vi "SpreadsheetFGV2_Improvements.vi"(0 "Student ID":i32, 1 "State Options":T4, 2 "Camera Name":refnum<k21> caption="IMAQdx Session", 5 "Message Ref":refnum<vi>, 9 "Front Panel References":refnum<vi>[](array[refnum]), 11 "Error In":errorcluster) -> (3 "Time Stamp Out":timestamp=timestamp(3628529847.18708 s since 1904-01-01), 4 "Message":string="Shut Down", 6 "Names":string[](array[string]), 8 "Output 2D Data":string[][](array[string])=[["Full Name", "Check In", "Check Out", "Checked In?", "Hours", "Minutes", "Seconds", "Total Seconds", "Col1", "Col2", "Col3", "Record ID (ref)", "Related Season Log"], ["Aden Lok", "", "", "FALSE", "", "", "", "", "0", "0", "0", "167", "239"], ["Aidan Egan", "", "", "FALSE", "", "", "", "", "0", "0", "0", "12", "240"], ["Alejandro Magadan", "12/24/2018 3:47:18 PM", "12/24/2018 3:53:19 PM", "FALSE", "15", "47", "18", "361", "0", "0", "0", "166", "241"], ["Alessandro Carleton", "", "", "FALSE", "", "", "", "", "0", "0", "0", "165", "242"], ["Amaan Ali", "", "", "FALSE", "", "", "", "", "0", "0", "0", "168", "243"], ["An Ngo", "", "", "FALSE", "", "", "", "", "0", "0", "0", "163", "244"], ["Avery Jennings", "", "", "FALSE", "", "", "", "", "0", "0", "0", "102", "245"], ["Brendan Webb", "12/24/2018 3:39:05 PM", "12/24/2018 3:53:19 PM", "FALSE", "15", "39", "05", "854", "0", "0", "0", "33", "246"], ["Brendan Byrne", "12/24/2018 3:47:17 PM", "12/24/2018 3:53:19 PM", "FALSE", "15", "47", "17", "362", "0", "0", "0", "169", "247"], ["Charles Jacobson", "12/24/2018 3:47:12 PM", "12/24/2018 3:48:43 PM", "FALSE", "15", "47", "12", "91", "0", "0", "0", "110", "248"], ["Chase Thomas", "", "", "FALSE", "", "", "", "", "0", "0", "0", "24", "249"], ["Christian Davis", "", "", "FALSE", "", "", "", "", "0", "0", "0", "171", "250"], ["Christopher Keith", "", "", "FALSE", "", "", "", "", "0", "0", "0", "170", "251"], ["Colman Gillis", "", "", "FALSE", "", "", "", "", "0", "0", "0", "62", "252"], ["Daniel Murtagh", "12/24/2018 3:38:36 PM", "12/24/2018 3:53:19 PM", "FALSE", "15", "38", "36", "883", "0", "0", "0", "173", "253"], ["Daniel Politano", "", "", "FALSE", "", "", "", "", "0", "0", "0", "175", "254"], ["Donovan Moore", "", "", "FALSE", "", "", "", "", "0", "0", "0", "174", "255"], ["Dyllan Bui", "", "", "FALSE", "", "", "", "", "0", "0", "0", "172", "256"], ["Henry Synnott", "", "", "FALSE", "", "", "", "", "0", "0", "0", "176", "257"], ["Huy GIang", "12/24/2018 3:47:20 PM", "12/24/2018 3:53:19 PM", "FALSE", "15", "47", "20", "359", "0", "0", "0", "177", "258"], ["Isaiah Jean-Fontaine", "", "", "FALSE", "", "", "", "", "0", "0", "0", "178", "259"], ["Jack Duggan", "", "", "FALSE", "", "", "", "", "0", "0", "0", "11", "260"], ["Jack Morris", "", "", "FALSE", "", "", "", "", "0", "0", "0", "181", "261"], ["Jake Monahan", "", "", "FALSE", "", "", "", "", "0", "0", "0", "189", "262"], ["James McEneaney", "", "", "FALSE", "", "", "", "", "0", "0", "0", "180", "263"], ["Jason Murray", "", "", "FALSE", "", "", "", "", "0", "0", "0", "16", "264"], ["Javed Brathwaite", "12/24/2018 3:39:10 PM", "12/24/2018 3:41:41 PM", "FALSE", "15", "39", "10", "151", "0", "0", "0", "72", "265"], ["Jay Siegfried", "", "", "FALSE", "", "", "", "", "0", "0", "0", "73", "266"], ["Jeffrey Chen", "", "", "FALSE", "", "", "", "", "0", "0", "0", "179", "267"], ["Karsten Patzer", "", "12/24/2018 3:53:19 PM", "FALSE", "", "", "", "57199", "0", "0", "0", "182", "268"], ["Liam Walsh", "", "", "FALSE", "", "", "", "", "0", "0", "0", "134", "269"], ["Lucas Hurley", "", "", "FALSE", "", "", "", "", "0", "0", "0", "183", "270"], ["Luke Reid", "", "", "FALSE", "", "", "", "", "0", "0", "0", "93", "271"], ["Maxwell Malamut", "", "", "FALSE", "", "", "", "", "0", "0", "0", "133", "272"], ["Nicholas Hurley", "", "", "FALSE", "", "", "", "", "0", "0", "0", "121", "273"], ["Philip Byrne", "", "", "FALSE", "", "", "", "", "0", "0", "0", "184", "274"], ["Praveen Kalva", "", "", "FALSE", "", "", "", "", "0", "0", "0", "185", "275"], ["Rohan Joshi", "", "", "FALSE", "", "", "", "", "0", "0", "0", "84", "276"], ["Samuel Danby", "", "", "FALSE", "", "", "", "", "0", "0", "0", "9", "277"], ["Thomas Potts", "", "", "FALSE", "", "", "", "", "0", "0", "0", "111", "278"], ["Timmy Tran", "", "", "FALSE", "", "", "", "", "0", "0", "0", "186", "279"], ["Willem Lenig", "", "", "FALSE", "", "", "", "", "0", "0", "0", "188", "280"], ["William Lau", "", "", "FALSE", "", "", "", "", "0", "0", "0", "187", "281"]], 10 "Checked In?":bool, 12 "Cat Points":i32, 13 "Image Out":T2(plugin-control), 14 "Elapsed Time":dbl, 15 "Error Out":errorcluster)   [LabVIEW 2018]
uses:
  Controls/CSVFGVStates.ctl
  <vilib>/userdefined/High Color/IMAQdx.ctl
  Controls/SpreadsheetColumns.ctl
  Controls/ClockType.ctl
  <vilib>/Utility/file.llb/Write Delimited Spreadsheet (string).vi
  <vilib>/Utility/file.llb/Read Delimited Spreadsheet (string).vi
  <vilib>/vision/driver/NI_Vision_Acquisition_Software.lvlib
panel:
  out "IDs":string[](array[string])
  out "headers":string
  out "body":string
  out "Camera Information Array":T1(array[cluster])=[{"Type"=3, "Version"=2, "Flags"=1, "SerialNumberHigh"=2886719754, "SerialNumberLow"=3015254064, "BusType"=1685284983, "InterfaceName"="cam2", "VendorName"="Microsoft® LifeCam Studio(TM)", "ModelName"="", "CameraFileName"="Microsoft® LifeCam Studio(TM)  (#AC0FD90AB3B92030).icd", "CameraAttributeURL"=""}] {"BusType" format="%x"; "SerialNumberLow" format="%.0x"; "SerialNumberHigh" format="%.0x"}
  out "Table List":string[][](array[string])=[["Full Name", "Check In", "Check Out", "Checked In?", "Hours", "Minutes", "Seconds", "Total Seconds", "Col1", "Col2", "Col3", "Record ID (ref)", "Related Season Log"], ["Aden Lok", "", "", "FALSE", "", "", "", "", "0", "0", "0", "167", "239"], ["Aidan Egan", "", "", "FALSE", "", "", "", "", "0", "0", "0", "12", "240"], ["Alejandro Magadan", "12/24/2018 3:47:18 PM", "12/24/2018 3:53:19 PM", "FALSE", "15", "47", "18", "361", "0", "0", "0", "166", "241"], ["Alessandro Carleton", "", "", "FALSE", "", "", "", "", "0", "0", "0", "165", "242"], ["Amaan Ali", "", "", "FALSE", "", "", "", "", "0", "0", "0", "168", "243"], ["An Ngo", "", "", "FALSE", "", "", "", "", "0", "0", "0", "163", "244"], ["Avery Jennings", "", "", "FALSE", "", "", "", "", "0", "0", "0", "102", "245"], ["Brendan Webb", "12/24/2018 3:39:05 PM", "12/24/2018 3:53:19 PM", "FALSE", "15", "39", "05", "854", "0", "0", "0", "33", "246"], ["Brendan Byrne", "12/24/2018 3:47:17 PM", "12/24/2018 3:53:19 PM", "FALSE", "15", "47", "17", "362", "0", "0", "0", "169", "247"], ["Charles Jacobson", "12/24/2018 3:47:12 PM", "12/24/2018 3:48:43 PM", "FALSE", "15", "47", "12", "91", "0", "0", "0", "110", "248"], ["Chase Thomas", "", "", "FALSE", "", "", "", "", "0", "0", "0", "24", "249"], ["Christian Davis", "", "", "FALSE", "", "", "", "", "0", "0", "0", "171", "250"], ["Christopher Keith", "", "", "FALSE", "", "", "", "", "0", "0", "0", "170", "251"], ["Colman Gillis", "", "", "FALSE", "", "", "", "", "0", "0", "0", "62", "252"], ["Daniel Murtagh", "12/24/2018 3:38:36 PM", "12/24/2018 3:53:19 PM", "FALSE", "15", "38", "36", "883", "0", "0", "0", "173", "253"], ["Daniel Politano", "", "", "FALSE", "", "", "", "", "0", "0", "0", "175", "254"], ["Donovan Moore", "", "", "FALSE", "", "", "", "", "0", "0", "0", "174", "255"], ["Dyllan Bui", "", "", "FALSE", "", "", "", "", "0", "0", "0", "172", "256"], ["Henry Synnott", "", "", "FALSE", "", "", "", "", "0", "0", "0", "176", "257"], ["Huy GIang", "12/24/2018 3:47:20 PM", "12/24/2018 3:53:19 PM", "FALSE", "15", "47", "20", "359", "0", "0", "0", "177", "258"], ["Isaiah Jean-Fontaine", "", "", "FALSE", "", "", "", "", "0", "0", "0", "178", "259"], ["Jack Duggan", "", "", "FALSE", "", "", "", "", "0", "0", "0", "11", "260"], ["Jack Morris", "", "", "FALSE", "", "", "", "", "0", "0", "0", "181", "261"], ["Jake Monahan", "", "", "FALSE", "", "", "", "", "0", "0", "0", "189", "262"], ["James McEneaney", "", "", "FALSE", "", "", "", "", "0", "0", "0", "180", "263"], ["Jason Murray", "", "", "FALSE", "", "", "", "", "0", "0", "0", "16", "264"], ["Javed Brathwaite", "12/24/2018 3:39:10 PM", "12/24/2018 3:41:41 PM", "FALSE", "15", "39", "10", "151", "0", "0", "0", "72", "265"], ["Jay Siegfried", "", "", "FALSE", "", "", "", "", "0", "0", "0", "73", "266"], ["Jeffrey Chen", "", "", "FALSE", "", "", "", "", "0", "0", "0", "179", "267"], ["Karsten Patzer", "", "12/24/2018 3:53:19 PM", "FALSE", "", "", "", "57199", "0", "0", "0", "182", "268"], ["Liam Walsh", "", "", "FALSE", "", "", "", "", "0", "0", "0", "134", "269"], ["Lucas Hurley", "", "", "FALSE", "", "", "", "", "0", "0", "0", "183", "270"], ["Luke Reid", "", "", "FALSE", "", "", "", "", "0", "0", "0", "93", "271"], ["Maxwell Malamut", "", "", "FALSE", "", "", "", "", "0", "0", "0", "133", "272"], ["Nicholas Hurley", "", "", "FALSE", "", "", "", "", "0", "0", "0", "121", "273"], ["Philip Byrne", "", "", "FALSE", "", "", "", "", "0", "0", "0", "184", "274"], ["Praveen Kalva", "", "", "FALSE", "", "", "", "", "0", "0", "0", "185", "275"], ["Rohan Joshi", "", "", "FALSE", "", "", "", "", "0", "0", "0", "84", "276"], ["Samuel Danby", "", "", "FALSE", "", "", "", "", "0", "0", "0", "9", "277"], ["Thomas Potts", "", "", "FALSE", "", "", "", "", "0", "0", "0", "111", "278"], ["Timmy Tran", "", "", "FALSE", "", "", "", "", "0", "0", "0", "186", "279"], ["Willem Lenig", "", "", "FALSE", "", "", "", "", "0", "0", "0", "188", "280"], ["William Lau", "", "", "FALSE", "", "", "", "", "0", "0", "0", "187", "281"]]
  out "Table List":string[][](array[string])=[["Full Name", "Check In", "Check Out", "Checked In?", "Hours", "Minutes", "Seconds", "Total Seconds", "Col1", "Col2", "Col3", "Record ID (ref)", "Related Season Log"], ["Aden Lok", "", "", "FALSE", "", "", "", "", "0", "0", "0", "167", "239"], ["Aidan Egan", "", "", "FALSE", "", "", "", "", "0", "0", "0", "12", "240"], ["Alejandro Magadan", "12/24/2018 3:47:18 PM", "", "TRUE", "15", "47", "18", "", "0", "0", "0", "166", "241"], ["Alessandro Carleton", "", "", "FALSE", "", "", "", "", "0", "0", "0", "165", "242"], ["Amaan Ali", "", "", "FALSE", "", "", "", "", "0", "0", "0", "168", "243"], ["An Ngo", "", "", "FALSE", "", "", "", "", "0", "0", "0", "163", "244"], ["Avery Jennings", "", "", "FALSE", "", "", "", "", "0", "0", "0", "102", "245"], ["Brendan Webb", "12/24/2018 3:39:05 PM", "", "TRUE", "15", "39", "05", "", "0", "0", "0", "33", "246"], ["Brendan Byrne", "12/24/2018 3:47:17 PM", "", "TRUE", "15", "47", "17", "", "0", "0", "0", "169", "247"], ["Charles Jacobson", "12/24/2018 3:47:12 PM", "", "TRUE", "15", "47", "12", "", "0", "0", "0", "110", "248"], ["Chase Thomas", "", "", "FALSE", "", "", "", "", "0", "0", "0", "24", "249"], ["Christian Davis", "", "", "FALSE", "", "", "", "", "0", "0", "0", "171", "250"], ["Christopher Keith", "", "", "FALSE", "", "", "", "", "0", "0", "0", "170", "251"], ["Colman Gillis", "", "", "FALSE", "", "", "", "", "0", "0", "0", "62", "252"], ["Daniel Murtagh", "12/24/2018 3:38:36 PM", "", "TRUE", "15", "38", "36", "", "0", "0", "0", "173", "253"], ["Daniel Politano", "", "", "FALSE", "", "", "", "", "0", "0", "0", "175", "254"], ["Donovan Moore", "", "", "FALSE", "", "", "", "", "0", "0", "0", "174", "255"], ["Dyllan Bui", "", "", "FALSE", "", "", "", "", "0", "0", "0", "172", "256"], ["Henry Synnott", "", "", "FALSE", "", "", "", "", "0", "0", "0", "176", "257"], ["Huy GIang", "", "", "FALSE", "", "", "", "", "0", "0", "0", "177", "258"], ["Isaiah Jean-Fontaine", "", "", "FALSE", "", "", "", "", "0", "0", "0", "178", "259"], ["Jack Duggan", "", "", "FALSE", "", "", "", "", "0", "0", "0", "11", "260"], ["Jack Morris", "", "", "FALSE", "", "", "", "", "0", "0", "0", "181", "261"], ["Jake Monahan", "", "", "FALSE", "", "", "", "", "0", "0", "0", "189", "262"], ["James McEneaney", "", "", "FALSE", "", "", "", "", "0", "0", "0", "180", "263"], ["Jason Murray", "", "", "FALSE", "", "", "", "", "0", "0", "0", "16", "264"], ["Javed Brathwaite", "12/24/2018 3:39:10 PM", "12/24/2018 3:41:41 PM", "FALSE", "15", "39", "10", "151", "0", "0", "0", "72", "265"], ["Jay Siegfried", "", "", "FALSE", "", "", "", "", "0", "0", "0", "73", "266"], ["Jeffrey Chen", "", "", "FALSE", "", "", "", "", "0", "0", "0", "179", "267"], ["Karsten Patzer", "", "", "TRUE", "", "", "", "", "0", "0", "0", "182", "268"], ["Liam Walsh", "", "", "FALSE", "", "", "", "", "0", "0", "0", "134", "269"], ["Lucas Hurley", "", "", "FALSE", "", "", "", "", "0", "0", "0", "183", "270"], ["Luke Reid", "", "", "FALSE", "", "", "", "", "0", "0", "0", "93", "271"], ["Maxwell Malamut", "", "", "FALSE", "", "", "", "", "0", "0", "0", "133", "272"], ["Nicholas Hurley", "", "", "FALSE", "", "", "", "", "0", "0", "0", "121", "273"], ["Philip Byrne", "", "", "FALSE", "", "", "", "", "0", "0", "0", "184", "274"], ["Praveen Kalva", "", "", "FALSE", "", "", "", "", "0", "0", "0", "185", "275"], ["Rohan Joshi", "", "", "FALSE", "", "", "", "", "0", "0", "0", "84", "276"], ["Samuel Danby", "", "", "FALSE", "", "", "", "", "0", "0", "0", "9", "277"], ["Thomas Potts", "", "", "FALSE", "", "", "", "", "0", "0", "0", "111", "278"], ["Timmy Tran", "", "", "FALSE", "", "", "", "", "0", "0", "0", "186", "279"], ["Willem Lenig", "", "", "FALSE", "", "", "", "", "0", "0", "0", "188", "280"], ["William Lau", "", "", "FALSE", "", "", "", "", "0", "0", "0", "187", "281"]]
  out "Session Out":T3="cam2"
  out "Checked In":string="FALSE"
  out "all rows":string[][](array[string])=[["Full Name", "Check In", "Check Out", "Checked In?", "Hours", "Minutes", "Seconds", "Total Seconds", "Col1", "Col2", "Col3", "Record ID (ref)", "Related Season Log"], ["Aden Lok", "", "", "FALSE", "", "", "", "", "0", "0", "0", "167", "239"], ["Aidan Egan", "", "", "FALSE", "", "", "", "", "0", "0", "0", "12", "240"], ["Alejandro Magadan", "12/24/2018 3:47:18 PM", "12/24/2018 3:53:19 PM", "FALSE", "15", "47", "18", "361", "0", "0", "0", "166", "241"], ["Alessandro Carleton", "", "", "FALSE", "", "", "", "", "0", "0", "0", "165", "242"], ["Amaan Ali", "", "", "FALSE", "", "", "", "", "0", "0", "0", "168", "243"], ["An Ngo", "", "", "FALSE", "", "", "", "", "0", "0", "0", "163", "244"], ["Avery Jennings", "", "", "FALSE", "", "", "", "", "0", "0", "0", "102", "245"], ["Brendan Webb", "12/24/2018 3:39:05 PM", "12/24/2018 3:53:19 PM", "FALSE", "15", "39", "05", "854", "0", "0", "0", "33", "246"], ["Brendan Byrne", "12/24/2018 3:47:17 PM", "12/24/2018 3:53:19 PM", "FALSE", "15", "47", "17", "362", "0", "0", "0", "169", "247"], ["Charles Jacobson", "12/24/2018 3:47:12 PM", "12/24/2018 3:48:43 PM", "FALSE", "15", "47", "12", "91", "0", "0", "0", "110", "248"], ["Chase Thomas", "", "", "FALSE", "", "", "", "", "0", "0", "0", "24", "249"], ["Christian Davis", "", "", "FALSE", "", "", "", "", "0", "0", "0", "171", "250"], ["Christopher Keith", "", "", "FALSE", "", "", "", "", "0", "0", "0", "170", "251"], ["Colman Gillis", "", "", "FALSE", "", "", "", "", "0", "0", "0", "62", "252"], ["Daniel Murtagh", "12/24/2018 3:38:36 PM", "12/24/2018 3:53:19 PM", "FALSE", "15", "38", "36", "883", "0", "0", "0", "173", "253"], ["Daniel Politano", "", "", "FALSE", "", "", "", "", "0", "0", "0", "175", "254"], ["Donovan Moore", "", "", "FALSE", "", "", "", "", "0", "0", "0", "174", "255"], ["Dyllan Bui", "", "", "FALSE", "", "", "", "", "0", "0", "0", "172", "256"], ["Henry Synnott", "", "", "FALSE", "", "", "", "", "0", "0", "0", "176", "257"], ["Huy GIang", "12/24/2018 3:47:20 PM", "12/24/2018 3:53:19 PM", "FALSE", "15", "47", "20", "359", "0", "0", "0", "177", "258"], ["Isaiah Jean-Fontaine", "", "", "FALSE", "", "", "", "", "0", "0", "0", "178", "259"], ["Jack Duggan", "", "", "FALSE", "", "", "", "", "0", "0", "0", "11", "260"], ["Jack Morris", "", "", "FALSE", "", "", "", "", "0", "0", "0", "181", "261"], ["Jake Monahan", "", "", "FALSE", "", "", "", "", "0", "0", "0", "189", "262"], ["James McEneaney", "", "", "FALSE", "", "", "", "", "0", "0", "0", "180", "263"], ["Jason Murray", "", "", "FALSE", "", "", "", "", "0", "0", "0", "16", "264"], ["Javed Brathwaite", "12/24/2018 3:39:10 PM", "12/24/2018 3:41:41 PM", "FALSE", "15", "39", "10", "151", "0", "0", "0", "72", "265"], ["Jay Siegfried", "", "", "FALSE", "", "", "", "", "0", "0", "0", "73", "266"], ["Jeffrey Chen", "", "", "FALSE", "", "", "", "", "0", "0", "0", "179", "267"], ["Karsten Patzer", "", "12/24/2018 3:53:19 PM", "FALSE", "", "", "", "57199", "0", "0", "0", "182", "268"], ["Liam Walsh", "", "", "FALSE", "", "", "", "", "0", "0", "0", "134", "269"], ["Lucas Hurley", "", "", "FALSE", "", "", "", "", "0", "0", "0", "183", "270"], ["Luke Reid", "", "", "FALSE", "", "", "", "", "0", "0", "0", "93", "271"], ["Maxwell Malamut", "", "", "FALSE", "", "", "", "", "0", "0", "0", "133", "272"], ["Nicholas Hurley", "", "", "FALSE", "", "", "", "", "0", "0", "0", "121", "273"], ["Philip Byrne", "", "", "FALSE", "", "", "", "", "0", "0", "0", "184", "274"], ["Praveen Kalva", "", "", "FALSE", "", "", "", "", "0", "0", "0", "185", "275"], ["Rohan Joshi", "", "", "FALSE", "", "", "", "", "0", "0", "0", "84", "276"], ["Samuel Danby", "", "", "FALSE", "", "", "", "", "0", "0", "0", "9", "277"], ["Thomas Potts", "", "", "FALSE", "", "", "", "", "0", "0", "0", "111", "278"], ["Timmy Tran", "", "", "FALSE", "", "", "", "", "0", "0", "0", "186", "279"], ["Willem Lenig", "", "", "FALSE", "", "", "", "", "0", "0", "0", "188", "280"], ["William Lau", "", "", "FALSE", "", "", "", "", "0", "0", "0", "187", "281"]]
  in  "Replacement":string
  in  "Student Names":i32(listbox)
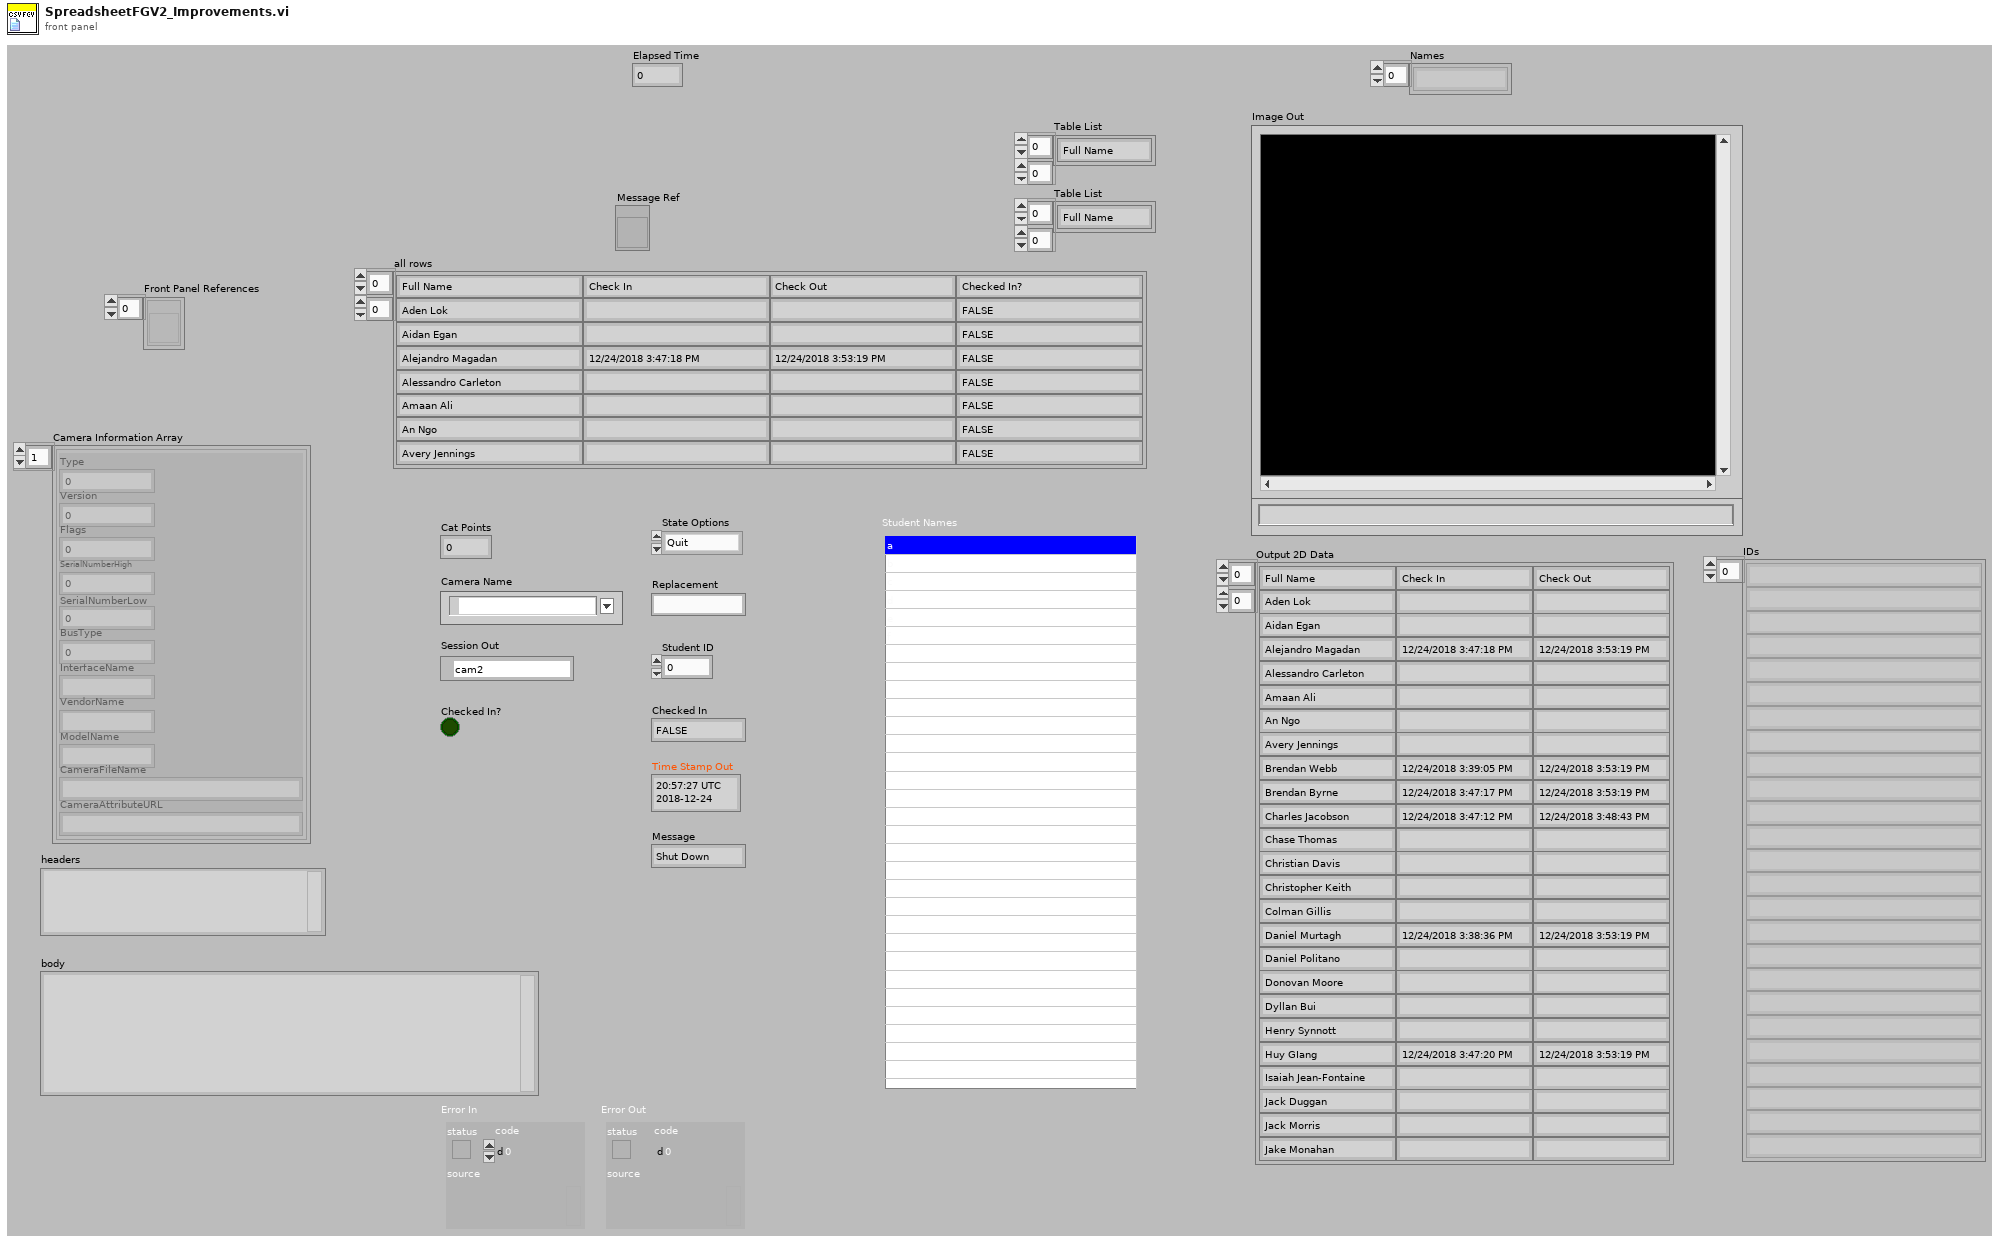
[diagram p1: front panel]
types:
  T1 = cluster{"Type":u32, "Version":u32, "Flags":u32, "SerialNumberHigh":u32, "SerialNumberLow":u32, "BusType":u32, "InterfaceName":string, "VendorName":string, "ModelName":string, "CameraFileName":string, "CameraAttributeURL":string}[]
  T2 = typedef "IMAQ Image.ctl" = refnum<image>
  T3 = typedef "IMAQdx.ctl" = refnum<k21>
  T4 = typedef "CSVFGVStates.ctl" = enum16{"Quit", "Init", "Sort", "Disable Camera", "Check In", "Check Out", "Check Status", "Read CSV", "Close Out"}
  T5 = typedef "SpreadsheetColumns.ctl" = enum16{"Email", "CheckIn", "CheckOut", "Checkin Flag", "Hours", "Minutes", "Seconds", "Total Seconds", "Cat Points"}
  T6 = cluster{"Checkin Flag":T5, "Check In":T5, "Hours":T5, "Minutes":T5, "Seconds":T5, "Check Out":T5, "Email":T5, "Total Seconds":T5}
  T7 = typedef "ClockType.ctl" = enum16{"Check In", "Close Out", "Check Out"}
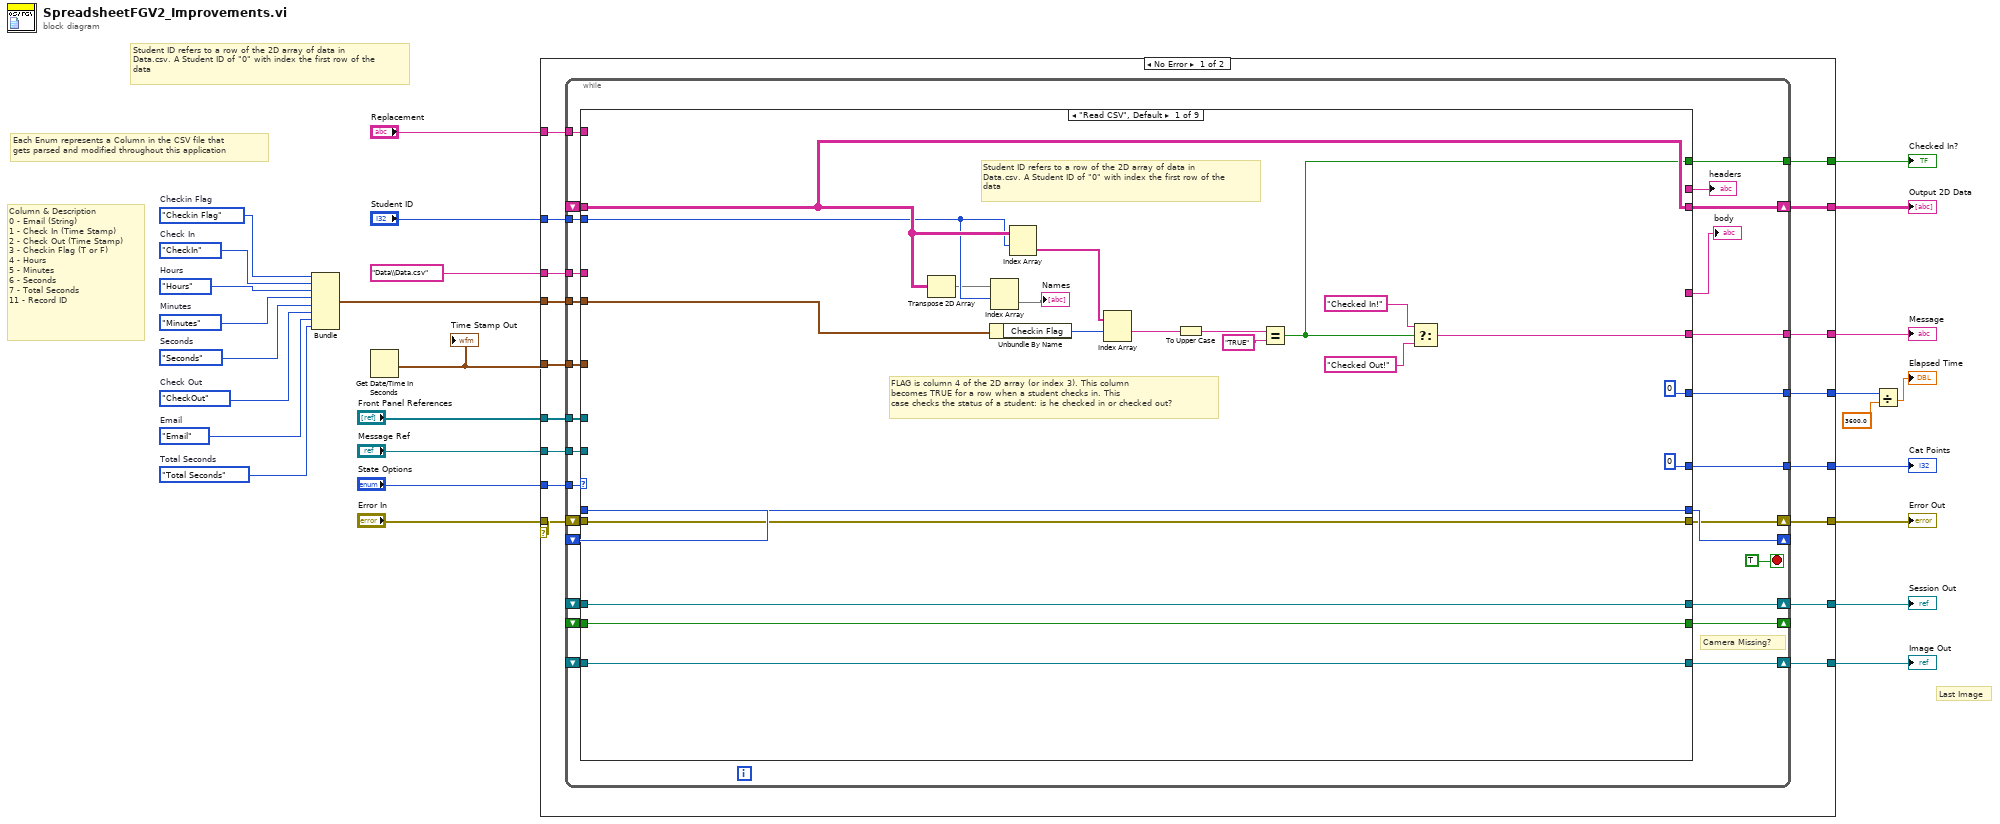
[diagram p0: block diagram]
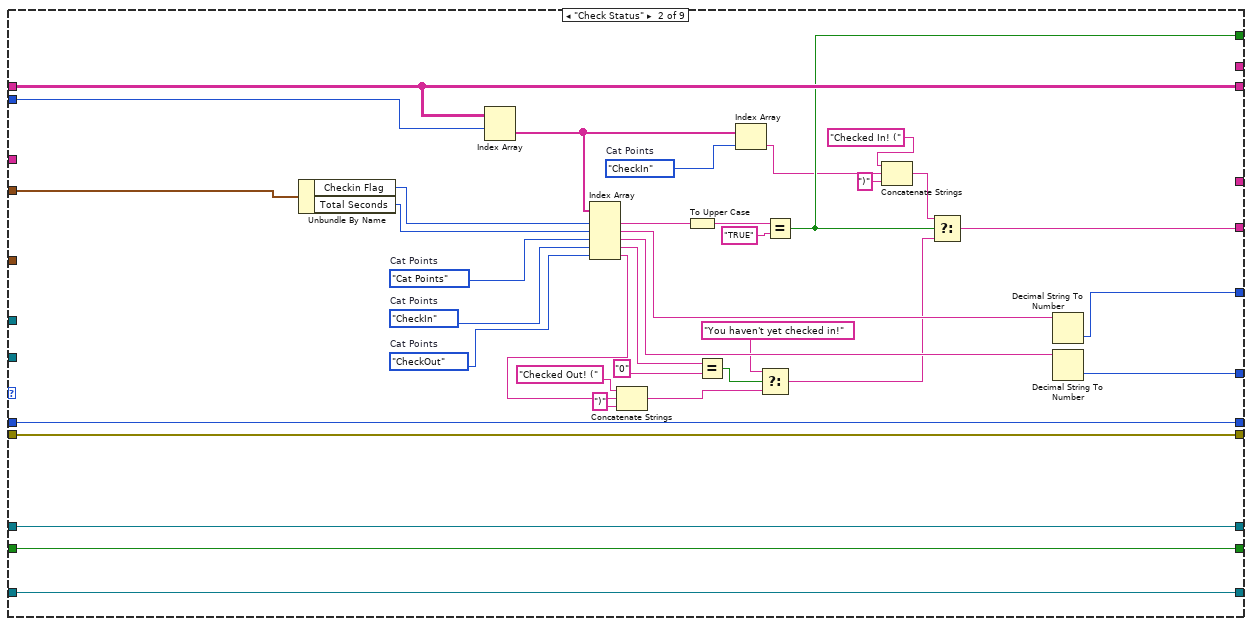
[diagram p2: hidden frame]
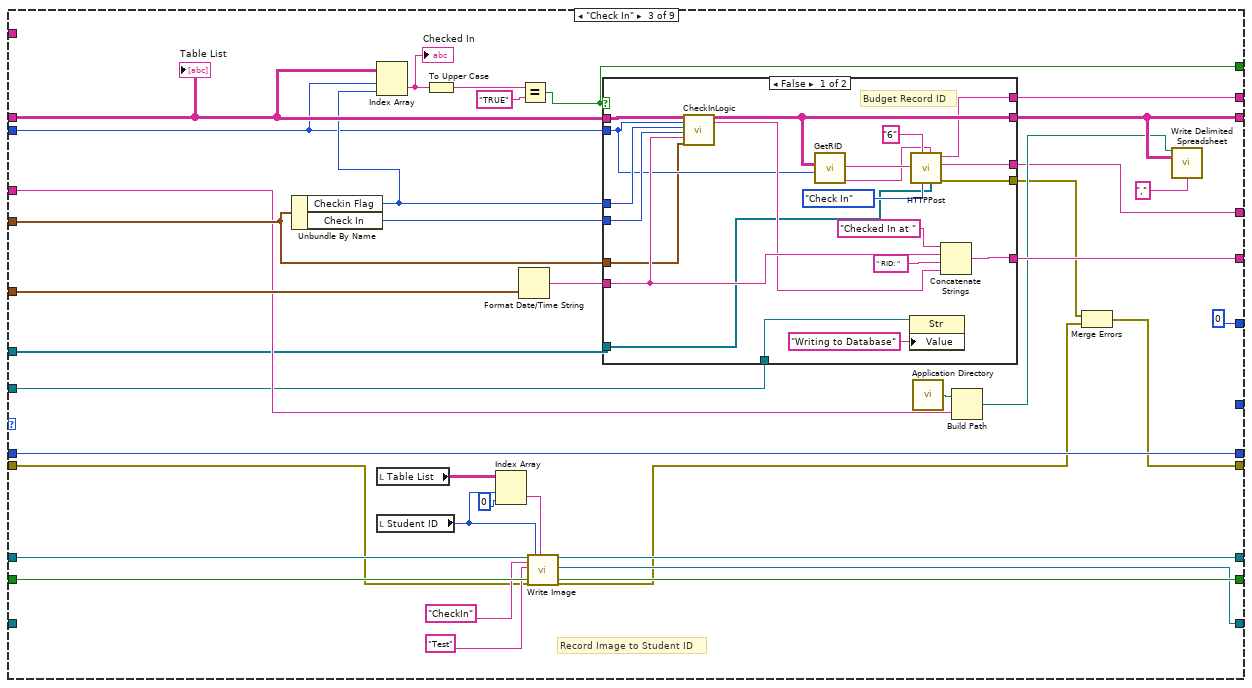
[diagram p3: hidden frame]
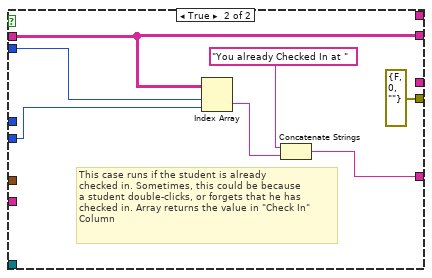
[diagram p4: hidden frame]
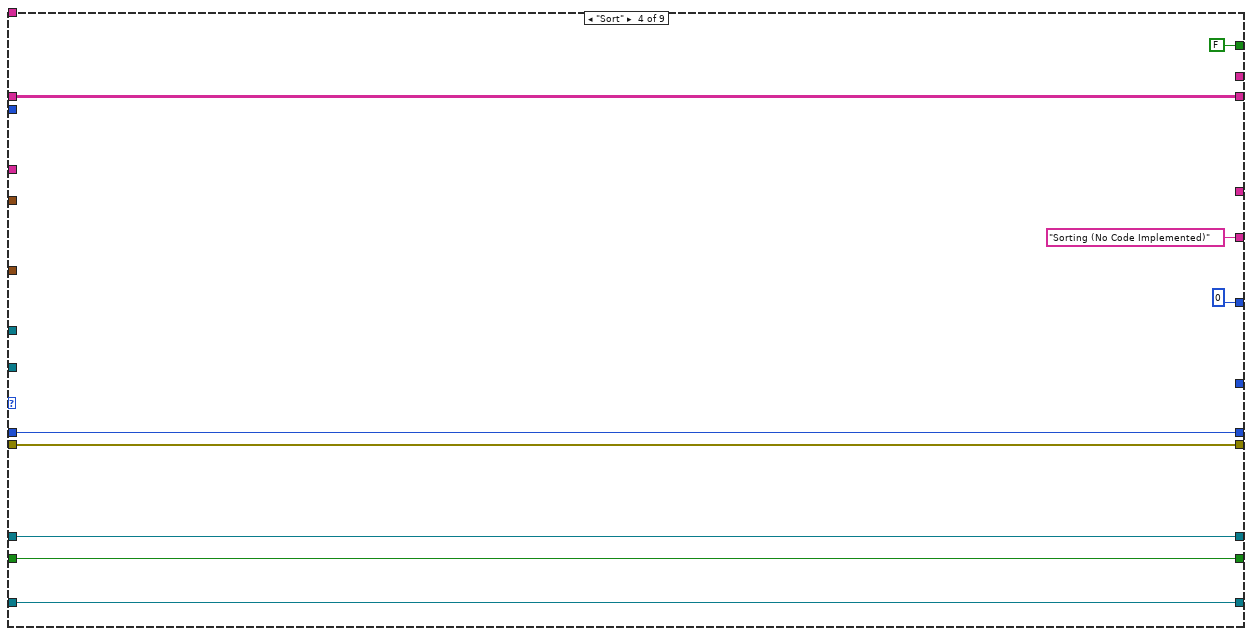
[diagram p5: hidden frame]
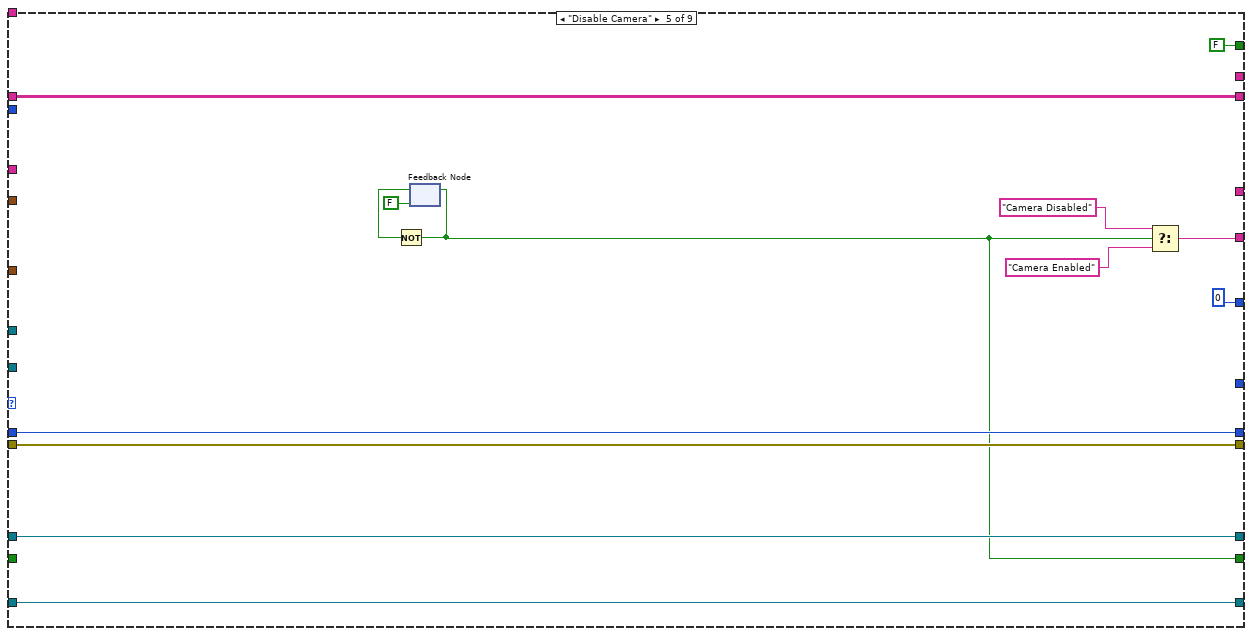
[diagram p6: hidden frame]
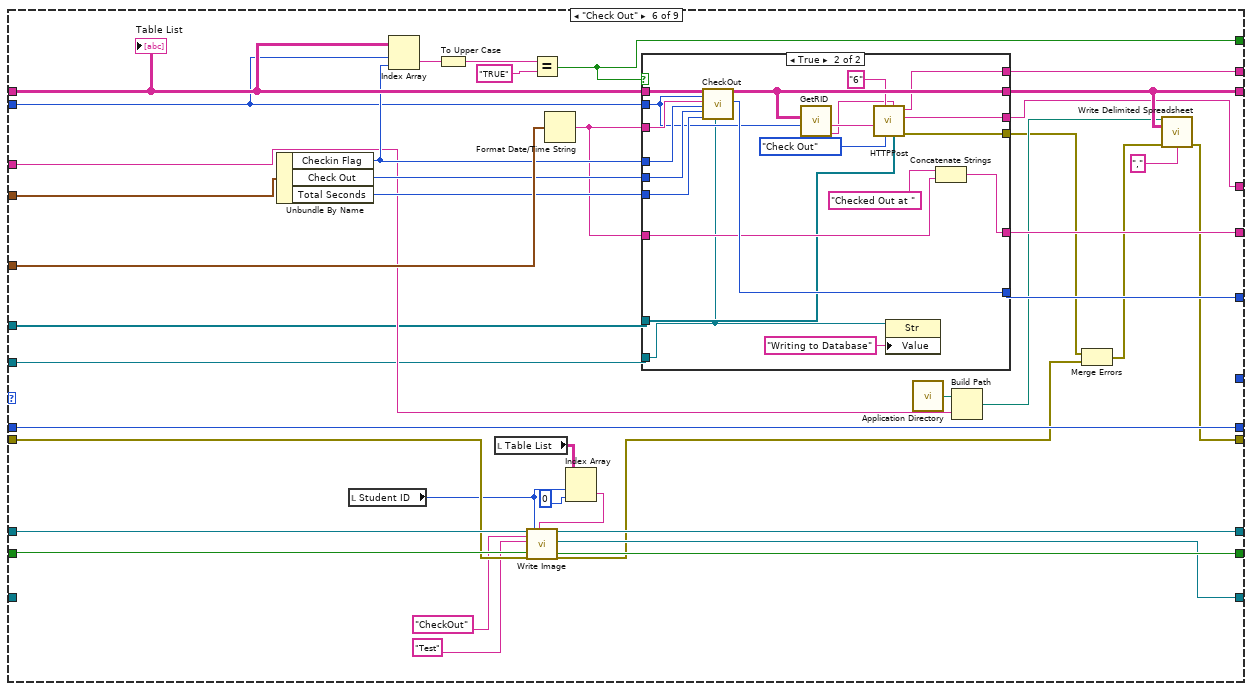
[diagram p7: hidden frame]
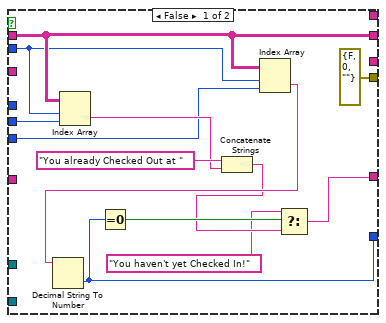
[diagram p8: hidden frame]
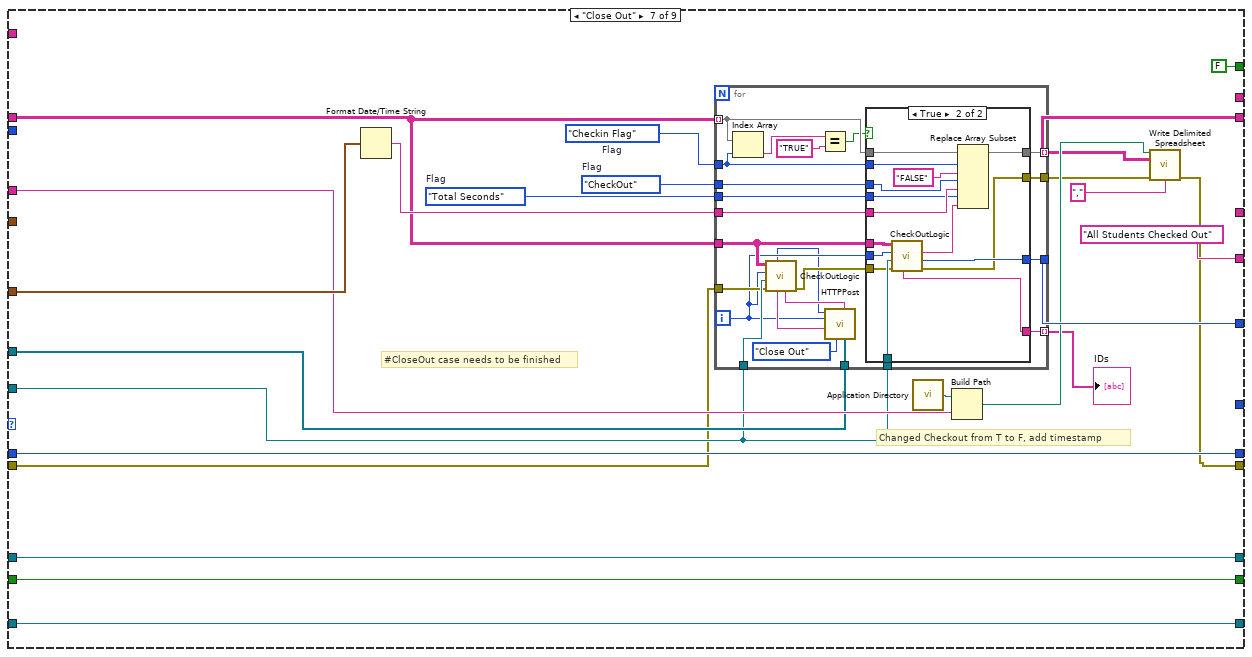
[diagram p9: hidden frame]
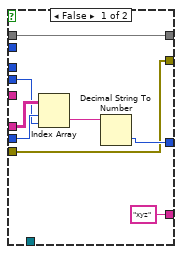
[diagram p10: hidden frame]
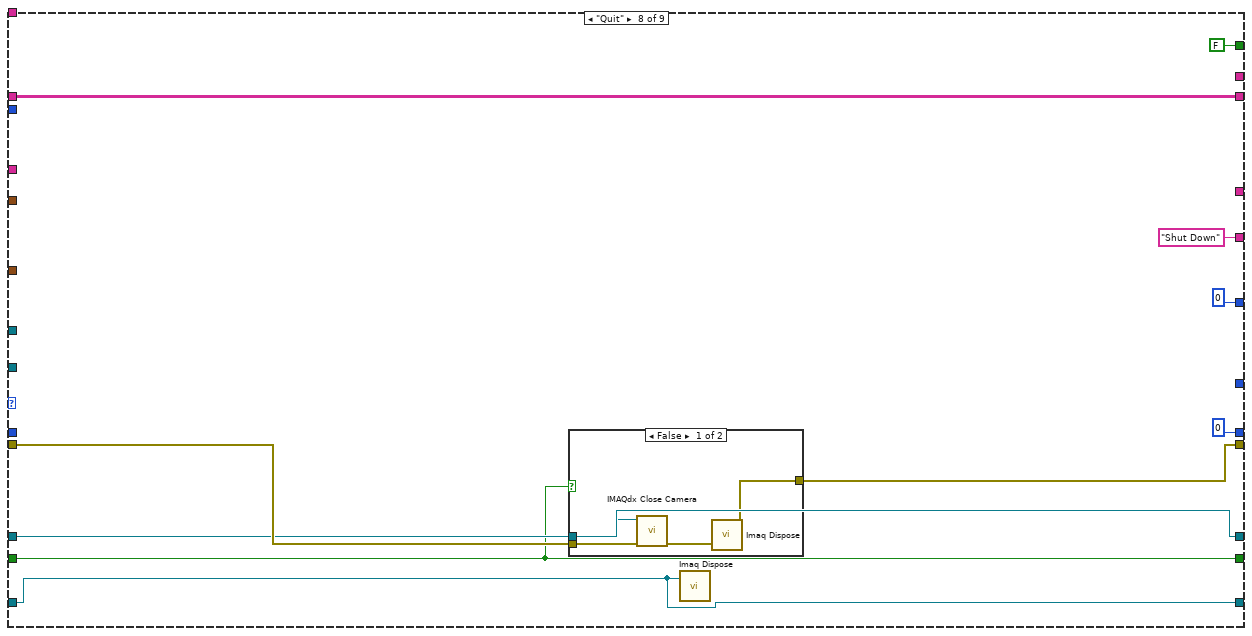
[diagram p11: hidden frame]
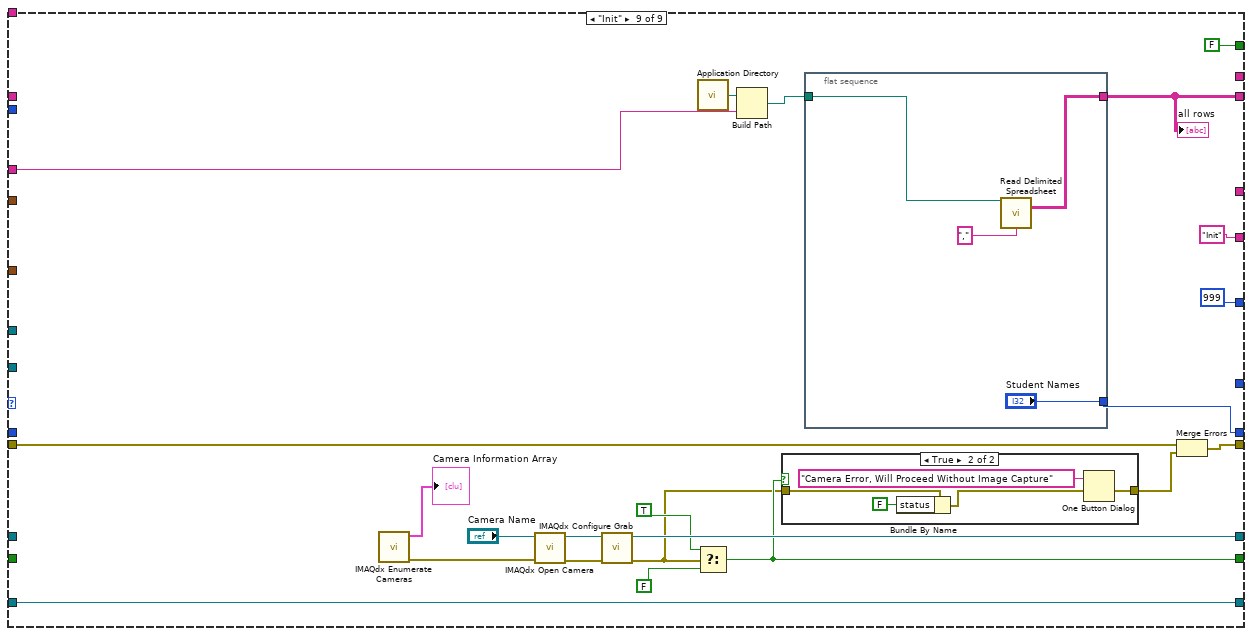
[diagram p13: hidden frame]
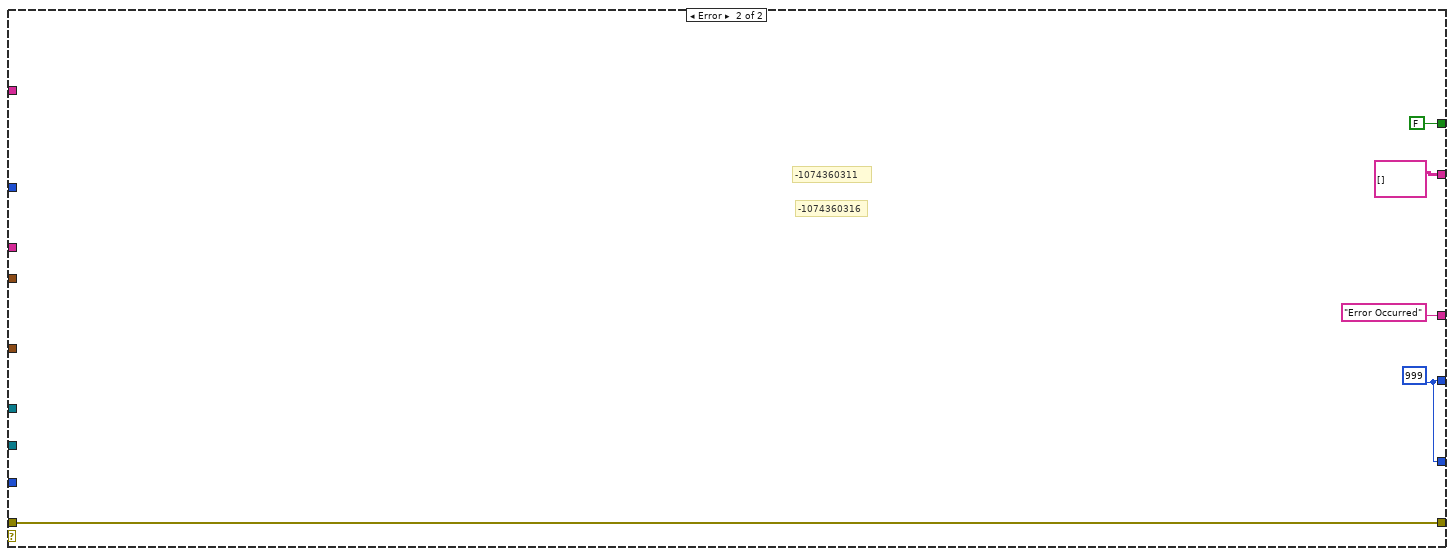
[diagram p15: hidden frame]
diagram:
  w12 = SpreadsheetColumns."Total Seconds"  # Total Seconds
  w13 = SpreadsheetColumns."Email"  # Email
  w14 = SpreadsheetColumns."CheckOut"  # Check Out
  w16 = SpreadsheetColumns."Seconds"  # Seconds
  w17 = SpreadsheetColumns."Minutes"  # Minutes
  w18 = SpreadsheetColumns."Hours"  # Hours
  w20 = SpreadsheetColumns."Checkin Flag"  # Checkin Flag
  w19 = SpreadsheetColumns."CheckIn"  # Check In
  # "Student ID refers to a row of the 2D array of data in \nData.csv. A Student ID of \"0\" with index the first row of the\ndata"
  # "Each Enum represents a Column in the CSV file that\ngets parsed and modified throughout this application"
  # "Last Image"
  # "Column & Description\n0 - Email (String)\n1 - Check In (Time Stamp)\n2 - Check Out (Time Stamp)\n3 - Checkin Flag (T or F)\n4 - Hours\n5 - Minutes\n6 - Seconds\n7 - Total Seconds\n11 - Record ID"
  n1 = Bundle("Checkin Flag"=w20, "Check In"=w19, "Hours"=w18, "Minutes"=w17, "Seconds"=w16, "Check Out"=w14, "Email"=w13, "Total Seconds"=w12) -> (w15:T6)  [unwired: 1 in]
  n2 = Get Date/Time In Seconds() -> (seconds since 1Jan1904=w9:timestamp)
  "Time Stamp Out" <- w9
  n3 = case shown="No Error" "Error In" {
    tunnel: "State Options" -> [w44 _]
    tunnel: "Error In" -> [w42 w406]
    tunnel: [w43 w406] -> w25
    tunnel: "Student ID" -> [w41 _]
    tunnel: w9 -> [w40 _]
    tunnel: "Replacement" -> [w39 _]
    tunnel: [w38 FALSE] -> w11
    tunnel: [w37 string[][] [] ("all rows")] -> w22
    tunnel: [w36 "Error Occurred" ("date/time string")] -> w21
    tunnel: [w35 w407] -> w6
    tunnel: w15 -> [w34 _]
    tunnel: "Data\\Data.csv" ("name or relative path") -> [w33 _]
    tunnel: [w32 w407] -> w8
    tunnel: [w31 _] -> w4
    tunnel: [w30 _] -> w3
    tunnel: "Front Panel References" -> [w29 _]
    tunnel: "Message Ref" -> [w28 _]
    frame No Error {
      n4 = while {
        shift-right: [w62] -> w37
        shift-left: _ -> [w57]
        tunnel: w44 -> [w70]
        shift-right: [w69] -> _
        shift-left: _ -> [w68]
        shift-right: [w67] -> w43
        shift-left: w42 -> [w66]
        tunnel: w41 -> [w65]
        tunnel: w40 -> [w64]
        tunnel: w39 -> [w63]
        tunnel: [w61] -> w38
        tunnel: [w60] -> w36
        tunnel: [w59] -> w35
        tunnel: w34 -> [w58]
        tunnel: w33 -> [w56]
        tunnel: [w55] -> w32
        shift-right: [w54] -> w31
        shift-left: _ -> [w53]
        shift-right: [w52] -> w30
        shift-left: _ -> [w51]
        shift-right: [w50] -> _
        shift-left: _ -> [w49]
        tunnel: w29 -> [w46]
        tunnel: w28 -> [w45]
        stop <- TRUE stop-if-true
        # "Camera Missing?"
        n5 = case shown="\"Read CSV\", Default" w70 {
          tunnel: w57 -> [w82 w123 w157 w198 w212 w249 w303 w369 _]
          tunnel: [w91 w128 w165 w202 w215 w254 w312 0 ("Student Names") w395] -> w69
          tunnel: w68 -> [w91 w128 w165 w202 w215 w254 w312 _ _]
          tunnel: [w92 w129 w134 w203 w216 w221 w290 w364 w377] -> w67
          tunnel: w66 -> [w92 w129 w144 w203 w216 w235 w291 w363 w378]
          tunnel: w65 -> [w81 w119 w151 _ _ w239 _ _ _]
          tunnel: w64 -> [_ _ w159 _ _ w253 w311 _ _]
          tunnel: w63 -> [_ _ _ _ _ _ _ _ _]
          tunnel: [w82 w123 w139 w198 w212 w227 w297 w369 w389] -> w62
          tunnel: [w78 w120 w156 FALSE FALSE w243 FALSE FALSE FALSE] -> w61
          tunnel: [w83 w124 w160 "Sorting (No Code Implemented)" ("date/time string") w207 w248 "All Students Checked Out" ("date/time string") "Shut Down" ("date/time string") "Init" ("date/time string")] -> w60
          tunnel: [0 ("Elapsed Seconds") w116 0 ("Elapsed Seconds") 0 ("Elapsed Seconds") 0 ("Elapsed Seconds") w247 w302 0 ("Elapsed Seconds") 999 ("Elapsed Seconds")] -> w59
          tunnel: w58 -> [w77 w122 w155 _ _ w246 _ _ _]
          tunnel: w56 -> [_ _ w154 _ _ w241 w307 _ w390]
          tunnel: [0 w113 _ _ _ _ _ _ _] -> w55
          tunnel: [w74 w95 w146 w197 w211 w237 w301 w362 w386] -> w54
          tunnel: w53 -> [w74 w95 w150 w197 w211 w238 w301 w362 _]
          tunnel: [w73 w94 w145 w196 w210 w234 w300 w360 w385] -> w52
          tunnel: w51 -> [w73 w94 _ w196 w210 _ w300 w360 w385]
          tunnel: [w72 w93 w149 w195 w204 w236 w299 w361 w382] -> w50
          tunnel: w49 -> [w72 w93 w149 w195 _ w236 w299 w361 _]
          tunnel: [_ _ w133 _ _ w219 _ _ _] -> w48
          tunnel: [_ _ w132 _ _ w220 _ _ _] -> w47
          tunnel: w46 -> [_ _ w131 _ _ w218 w294 _ _]
          tunnel: w45 -> [_ _ w130 _ _ w217 w293 _ _]
          frame "Read CSV", Default {
            # "FLAG is column 4 of the 2D array (or index 3). This column\nbecomes TRUE for a row when a student checks in. This\ncase checks the status of a student: is he checked in or checked out?"
            # "Student ID refers to a row of the 2D array of data in \nData.csv. A Student ID of \"0\" with index the first row of the\ndata"
            n6 = Transpose 2D Array(2D array=w82) -> (transposed array=w80:string[][])
            n7 = Unbundle By Name(w77) -> ("Checkin Flag"=w76:T5)
            n8 = Index Array(array=w80, index (row)=w81) -> (element=→"Names":string[])  [unwired: 1 in]
            n9 = Index Array(array=w82, index (row)=w81) -> (element=w86:string[])  [unwired: 1 in]
            n10 = Index Array(array=w86, index #1=w76) -> (element #1=w89:string)  [unwired: 1 in, 1 out]
            n11 = To Upper Case(1:w89) -> (0:w88:string)
            n12 = Equal?(x=w88, y="TRUE") -> (x = y?=w78:bool)
            n13 = Select(t="Checked In!" ("y"), s=w78, f="Checked Out!" ("y")) -> (s? t:f=w83:string)
          }
          frame "Check Status" {
            w101 = SpreadsheetColumns."CheckIn"  # Cat Points
            w100 = SpreadsheetColumns."CheckOut"  # Cat Points
            w112 = SpreadsheetColumns."CheckIn"  # Cat Points
            w115 = SpreadsheetColumns."Cat Points"  # Cat Points
            n14 = Unbundle By Name(w122) -> ("Checkin Flag"=w121:T5, "Total Seconds"=w118:T5)
            n15 = Index Array(array=w123, index (row)=w119) -> (element=w102:string[])  [unwired: 1 in]
            n16 = Index Array(array=w102, index #1=w121, index #2=w118, index #3=w115, index #4=w112, index #5=w100) -> (element #1=w127:string, element #2=w117:string, element #3=w114:string, element #4=w111:string, element #5=w104:string)
            n17 = Concatenate Strings("Checked Out! (" ("y"), w104, ")" ("string")) -> (w105:string)
            n18 = To Upper Case(1:w127) -> (0:w126:string)
            n19 = Equal?(x=w111, y="0") -> (x = y?=w109:bool)
            n20 = Index Array(array=w102, index=w101) -> (element=w98:string)
            n21 = Select(t="You haven't yet checked in!", s=w109, f=w105) -> (s? t:f=w108:string)
            n22 = Equal?(x=w126, y="TRUE") -> (x = y?=w120:bool)
            n23 = Concatenate Strings("Checked In! (" ("y"), w98, ")" ("string")) -> (w96:string)
            n24 = Select(t=w96, s=w120, f=w108) -> (s? t:f=w124:string)
            n25 = Decimal String To Number(string=w117) -> (number=w116:i32)  [unwired: 2 in, 1 out]
            n26 = Decimal String To Number(string=w114) -> (number=w113:i32)  [unwired: 2 in, 1 out]
          }
          frame "Check In" {
            # "Record Image to Student ID"
            n27 = Unbundle By Name(w155) -> ("Checkin Flag"=w153:T5, "Check In"=w158:T5)
            n28 = Index Array(array=w157, index (row)=w151, index (col)=w153) -> (element=w163:string)
            "Checked In" <- w163
            n29 = local read "Table List"() -> (w143:string[][])
            n30 = local read "Student ID"() -> (w142:i32)
            n31 = To Upper Case(1:w163) -> (0:w162:string)
            n32 = Index Array(array=w143, index (row)=w142, index (col)=0 ("disabled index (col)")) -> (element=w140:string)
            n33 = Format Date/Time String(seconds (now)=w159) -> (date/time string=w164:string)  [unwired: 2 in]
            n34 = Equal?(x=w162, y="TRUE") -> (x = y?=w156:bool)
            n35 = call "Write Image.vi"("Session In"=w150, "Folder"="CheckIn", "Temp Image Name"="Test" ("Image Name"), "Camera Missing?"=w149, "Error In"=w144, "Student ID"=w142, "Student Name"=w140) -> ("Session Out"=w146:T3, "Image Out"=w145:T2, "Error Out"=w135:errorcluster)  [unwired: 10 in]
            n36 = case shown="False" w156 {
              tunnel: w164 -> [w182 _]
              tunnel: [w178 w194] -> w139
              tunnel: w151 -> [w177 w193]
              tunnel: w157 -> [w185 w194]
              tunnel: [w186 w190] -> w160
              tunnel: w153 -> [w184 _]
              tunnel: w158 -> [w183 w189]
              tunnel: w155 -> [w171 _]
              tunnel: [w176 errorcluster {"status"=FALSE, "code"=0, "source"=""} ("error out")] -> w136
              tunnel: [w173 _] -> w133
              tunnel: [w172 _] -> w132
              tunnel: w131 -> [w170 _]
              tunnel: w130 -> [w168 _]
              frame False {
                # "Budget Record ID"
                n37 = call "CheckInLogic.vi"("all rows in"=w185, "Student ID"=w177, "Checkin Flag"=w184, "Check In"=w183, "date/time string"=w182, "Time Cluster"=w171) -> ("all rows out"=w178:string[][], "Student Record ID"=w180:string)  [unwired: 12 in]
                n38 = call "GetRID.vi"("Student ID in"=w177, "all rows in in"=w178) -> ("Season Log ID"=w167:string, "Record ID"=w179:string)  [unwired: 7 in]
                n39 = property class="Str"(reference=w168, "Value"="Writing to Database") -> ()  [unwired: 1 in, 2 out]
                n40 = call "HTTPPost.vi"("Front Panel References"=w170, "Season Log"=w167, "Clock Type"=ClockType."Check In", "Budget Year RID"="6", "Student RID"=w179) -> ("error out"=w176:errorcluster, "body"=w173:string, "headers"=w172:string)  [unwired: 4 in]
                n41 = Concatenate Strings("Checked In at " ("String"), w182, " RID: " ("string"), w180) -> (w186:string)
              }
              frame True {
                # "This case runs if the student is already \nchecked in. Sometimes, this could be because\na student double-clicks, or forgets that he has \nchecked in. Array returns the value in \"Check In\" \nColumn"
                n42 = Index Array(array=w194, index (row)=w193, index (col)=w189) -> (element=w191:string)
                n43 = Concatenate Strings("You already Checked In at " ("delimiter (\\t)"), w191) -> (w190:string)
              }
            }
            n44 = call <vilib>:"Application Directory.vi"() -> ("Application Directory"=w166:path)
            n45 = Build Path(base path=w166, name or relative path=w154) -> (appended path=w138:path)
            n46 = Merge Errors(w136, w135) -> (w134:errorcluster)
            n47 = call-poly <vilib>:"Write Delimited Spreadsheet.vi"("file path (dialog if empty)"=w138, "2D data"=w139, "delimiter (\\t)"="," ("delimiter (\\t)")) -> ()  [unwired: 11 in, 2 out]
            "Table List" <- w157
          }
          frame "Sort" {
          }
          frame "Disable Camera" {
            n48 = feedback #1(FALSE) -> (w205:bool)
            n49 = Not(x=w205) -> (.not. x?=w204:bool)
            n50 = feedback-in #1(w204) -> ()
            n51 = Select(t="Camera Disabled" ("date/time string"), s=w204, f="Camera Enabled" ("date/time string")) -> (s? t:f=w207:string)
          }
          frame "Check Out" {
            n52 = Unbundle By Name(w246) -> ("Checkin Flag"=w242:T5, "Check Out"=w244:T5, "Total Seconds"=w245:T5)
            n53 = local read "Student ID"() -> (w230:i32)
            n54 = Index Array(array=w249, index (row)=w239, index (col)=w242) -> (element=w252:string)
            n55 = To Upper Case(1:w252) -> (0:w251:string)
            n56 = local read "Table List"() -> (w231:string[][])
            n57 = Equal?(x=w251, y="TRUE") -> (x = y?=w243:bool)
            n58 = Format Date/Time String(seconds (now)=w253) -> (date/time string=w240:string)  [unwired: 2 in]
            n59 = Index Array(array=w231, index (row)=w230, index (col)=0 ("disabled index (col)")) -> (element=w228:string)
            n60 = call "Write Image.vi"("Session In"=w238, "Folder"="CheckOut", "Temp Image Name"="Test" ("Image Name"), "Camera Missing?"=w236, "Error In"=w235, "Student ID"=w230, "Student Name"=w228) -> ("Session Out"=w237:T3, "Image Out"=w234:T2, "Error Out"=w223:errorcluster)  [unwired: 10 in]
            n61 = case shown="True" w243 {
              tunnel: [w265 w279] -> w227
              tunnel: w239 -> [w264 w278]
              tunnel: w249 -> [w265 w287]
              tunnel: [w258 w289] -> w248
              tunnel: [w261 w282] -> w247
              tunnel: w245 -> [w263 w285]
              tunnel: w244 -> [w266 w286]
              tunnel: w242 -> [_ w284]
              tunnel: w240 -> [_ w283]
              tunnel: w240 -> [_ w281]
              tunnel: [errorcluster {"status"=FALSE, "code"=0, "source"=""} ("error out") w275] -> w224
              tunnel: [_ w274] -> w220
              tunnel: [_ w273] -> w219
              tunnel: w218 -> [_ w272]
              tunnel: w217 -> [_ w269]
              frame False {
                n62 = Index Array(array=w265, index (row)=w264, index (col)=w266) -> (element=w267:string)
                n63 = Concatenate Strings("You already Checked Out at " ("string"), w267) -> (w259:string)
                n64 = Index Array(array=w265, index (row)=w264, index (col)=w263) -> (element=w262:string)
                n65 = Decimal String To Number(string=w262) -> (number=w261:i32)  [unwired: 2 in, 1 out]
                n66 = Equal To 0?(x=w261) -> (x = 0?=w260:bool)
                n67 = Select(t="You haven't yet Checked In!", s=w260, f=w259) -> (s? t:f=w258:string)
              }
              frame True {
                n68 = call "CheckOut.vi"("Student List In"=w287, "Student ID"=w278, "date/time string"=w283, "Checkin Flag"=w284, "Check Out"=w286, "Total Seconds"=w285, "Message Ref"=w269) -> ("Student List Out"=w279:string[][], "Total Elapsed Time"=w282:i32)  [unwired: 11 in]
                n69 = call "GetRID.vi"("Student ID in"=w278, "all rows in in"=w279) -> ("Season Log ID"=w270:string, "Record ID"=w280:string)  [unwired: 7 in]
                n70 = call "HTTPPost.vi"("Front Panel References"=w272, "Season Log"=w270, "Clock Type"=ClockType."Check Out", "Budget Year RID"="6", "Student RID"=w280) -> ("error out"=w275:errorcluster, "body"=w273:string, "headers"=w274:string)  [unwired: 4 in]
                n71 = property class="Str"(reference=w269, "Value"="Writing to Database") -> ()  [unwired: 1 in, 2 out]
                n72 = Concatenate Strings("Checked Out at " ("string"), w281) -> (w289:string)
              }
            }
            n73 = call <vilib>:"Application Directory.vi"() -> ("Application Directory"=w255:path)
            n74 = Build Path(base path=w255, name or relative path=w241) -> (appended path=w225:path)
            n75 = Merge Errors(w224, w223) -> (w222:errorcluster)
            n76 = call-poly <vilib>:"Write Delimited Spreadsheet.vi"("file path (dialog if empty)"=w225, "2D data"=w227, "error in (no error)"=w222, "delimiter (\\t)"="," ("delimiter (\\t)")) -> ("error out"=w221:errorcluster)  [unwired: 10 in, 1 out]
            "Table List" <- w249
          }
          frame "Close Out" {
            w304 = SpreadsheetColumns."Total Seconds"  # Flag
            w305 = SpreadsheetColumns."CheckOut"  # Flag
            w306 = SpreadsheetColumns."Checkin Flag"  # Flag
            # "#CloseOut case needs to be finished"
            # "Changed Checkout from T to F, add timestamp"
            n77 = Format Date/Time String(seconds (now)=w311) -> (date/time string=w309:string)  [unwired: 2 in]
            n78 = for {
              tunnel: [w336] -> w297 mode=indexing
              tunnel: w303 -> [w331] mode=indexing
              tunnel: w309 -> [w335]
              tunnel: w306 -> [w330]
              tunnel: w305 -> [w334]
              tunnel: w304 -> [w333]
              tunnel: w303 -> [w322]
              tunnel: [w332] -> w302
              tunnel: [w326] -> w295 mode=indexing
              tunnel: w294 -> [w324]
              tunnel: w293 -> [w321]
              tunnel: w293 -> [w320]
              tunnel: w291 -> [w318]
              tunnel: [w316] -> w292
              i -> [w315]
              n79 = Index Array(array=w331, index=w330) -> (element=w329:string)
              n80 = call "CheckOutLogic.vi"("error in (no error)"=w318, "Message Ref"=w320, "Student ID"=w315, "Student List In"=w322) -> ("error out"=w317:errorcluster, "Season Log ID"=w323:string, "Record ID"=w319:string, "Student List Size"=w314:i32)  [unwired: 3 out]
              n81 = Equal?(x=w329, y="TRUE") -> (x = y?=w327:bool)
              n82 = call "HTTPPost.vi"("Front Panel References"=w324, "Season Log"=w323, "Clock Type"=ClockType."Close Out", "Student RID"=w319, "Iteration"=w315, "Student List Size"=w314) -> ()  [unwired: 3 in, 3 out]
              n83 = case shown="True" w327 {
                tunnel: [w344 w359] -> w336
                tunnel: w335 -> [_ w357]
                tunnel: w334 -> [_ w356]
                tunnel: w315 -> [w342 w355]
                tunnel: w333 -> [w341 w353]
                tunnel: w322 -> [w343 w352]
                tunnel: [w339 w351] -> w332
                tunnel: w331 -> [w344 w350]
                tunnel: w330 -> [_ w349]
                tunnel: ["xyz" ("Record ID") w347] -> w326
                tunnel: w321 -> [_ w348]
                tunnel: w317 -> [w337 w346]
                tunnel: [w337 w345] -> w316
                frame False {
                  n84 = Index Array(array=w343, index (row)=w342, index (col)=w341) -> (element=w340:string)
                  n85 = Decimal String To Number(string=w340) -> (number=w339:i32)  [unwired: 2 in, 1 out]
                }
                frame True {
                  n86 = call "CheckOutLogic.vi"("error in (no error)"=w346, "Message Ref"=w348, "Student ID"=w355, "Student List In"=w352) -> ("error out"=w345:errorcluster, "Total Elapsed Time"=w351:i32, "Total Seconds Out"=w354:string, "Record ID"=w347:string)  [unwired: 3 out]
                  n87 = Replace Array Subset(array=w350, new element #1="FALSE" ("new element/subarray"), index #1=w349, new element #2=w357, index #2=w356, new element #3=w354, index #3=w353) -> (w359:string[])
                }
              }
            }
            "IDs" <- w295
            n88 = call <vilib>:"Application Directory.vi"() -> ("Application Directory"=w313:path)
            n89 = Build Path(base path=w313, name or relative path=w307) -> (appended path=w298:path)
            n90 = call-poly <vilib>:"Write Delimited Spreadsheet.vi"("file path (dialog if empty)"=w298, "2D data"=w297, "error in (no error)"=w292, "delimiter (\\t)"="," ("delimiter (\\t)")) -> ("error out"=w290:errorcluster)  [unwired: 10 in, 1 out]
          }
          frame "Quit" {
            n91 = case shown="False" w361 {
              tunnel: [w372 w374] -> w364
              tunnel: w363 -> [w371 w374]
              tunnel: w362 -> [w370 _]
              frame False {
                n92 = call <vilib>:"IMAQdx Close Camera.vi"("error in"=w371, "Session In"=w370) -> ("error out"=w373:errorcluster)  [unwired: 9 out]
                n93 = call "Imaq Dispose"("error in (no error)"=w373) -> ("error out"=w372:errorcluster)  [unwired: 5 in]
              }
              frame True {
              }
            }
            n94 = call "Imaq Dispose"("Image"=w360) -> ()  [unwired: 5 in, 1 out]
          }
          frame "Init" {
            n95 = call <vilib>:"IMAQdx Enumerate Cameras.vi"() -> ("error out"=w380:errorcluster, "Camera Information Array"=→"Camera Information Array":T1)  [unwired: 10 in]
            n96 = call <vilib>:"IMAQdx Open Camera.vi"("error in"=w380, "Session In"="Camera Name") -> ("error out"=w379:errorcluster, "Session Out"=w388:T3)  [unwired: 1 in, 7 out]
            n97 = call <vilib>:"IMAQdx Configure Grab.vi"("error in"=w379, "Session In"=w388) -> ("error out"=w376:errorcluster, "Session Out"=w386:T3)  [unwired: 8 out]
            n98 = call <vilib>:"Application Directory.vi"() -> ("Application Directory"=w396:path)
            n99 = Select(t=TRUE, s=w376, f=FALSE) -> (s? t:f=w382:bool)
            n100 = Build Path(base path=w396, name or relative path=w390) -> (appended path=w394:path)
            n101 = case shown="True" w382 {
              tunnel: w376 -> [w397 w400]
              tunnel: [w397 w398] -> w375
              frame False {
              }
              frame True {
                n102 = Bundle By Name(cluster=w400, "status"=FALSE) -> (w398:errorcluster)
                n103 = One Button Dialog(message="Camera Error, Will Proceed Without Image Capture") -> ()  [unwired: 1 in, 1 out]
              }
            }
            n104 = flat-sequence {
              tunnel: w394 -> [w404]
              tunnel: [w403] -> w389
              tunnel: ["Student Names"] -> w395
              frame #0 {
                n105 = call-poly <vilib>:"Read Delimited Spreadsheet.vi"("file path (dialog if empty)"=w404, "delimiter (\\t)"="," ("delimiter (\\t)")) -> ("all rows"=w403:string[][])  [unwired: 8 in, 5 out]
              }
            }
            n106 = Merge Errors(w378, w375) -> (w377:errorcluster)
            "all rows" <- w389
          }
        }
        "headers" <- w47
        "body" <- w48
      }
    }
    frame Error {
      w407 = 999 ("Elapsed Seconds")
      # "-1074360316"
      # "-1074360311"
    }
  }
  "Error Out" <- w25
  "Checked In?" <- w11
  "Output 2D Data" <- w22
  "Message" <- w21
  "Cat Points" <- w8
  "Session Out" <- w4
  "Image Out" <- w3
  n107 = Divide(x=w6, y=3600.0) -> (x/y=→"Elapsed Time":dbl)
